vi "JSON to Name Value Pairs.vi"(10 "Message":string) -> (2 "Name Value Pairs":string[][](array[string]))   [LabVIEW 2018]
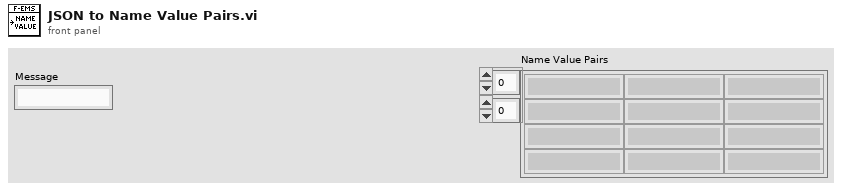
[diagram p1: front panel]
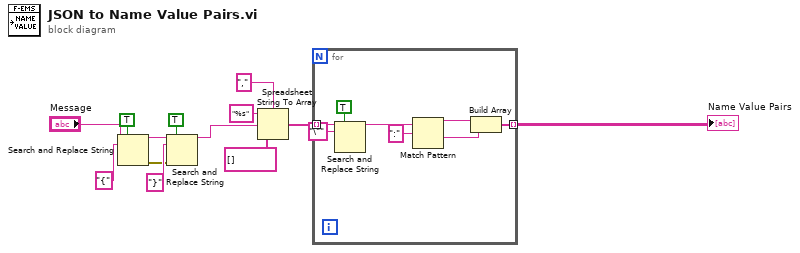
[diagram p0: block diagram]
diagram:
  n1 = Search and Replace String(replace all?=TRUE ("replace all? (F)"), input string="Message", search string="{") -> (result string=w2:string, error out=w3:errorcluster)  [unwired: 5 in, 2 out]
  n2 = Search and Replace String(replace all?=TRUE ("replace all? (F)"), input string=w2, search string="}", error in=w3) -> (result string=w1:string)  [unwired: 4 in, 3 out]
  n3 = Spreadsheet String To Array(delimiter (Tab)=",", format string="%s", spreadsheet string=w1, array type (2D Dbl)=string[] [] ("Name Value Pairs 2")) -> (array=w11:string[])
  n4 = for {
    tunnel: w11 -> [w20] mode=indexing
    tunnel: [w15] -> w10 mode=indexing
    n5 = Search and Replace String(replace all?=TRUE ("replace all? (F)"), input string=w20, search string="\"") -> (result string=w19:string)  [unwired: 5 in, 3 out]
    n6 = Match Pattern(string=w19, regular expression=":") -> (before substring=w17:string, after substring=w16:string)  [unwired: 1 in, 2 out]
    n7 = Build Array(w17, w16) -> (w15:string[])
  }
  "Name Value Pairs" <- w10
